vi "PollReceiveQueueNoSemaphore.vi"(8 "error in (no error)":errorcluster, 10 "waiting time ms (-1: forever)":i32=10, 11 "queue cluster":T1) -> (1 "receive queue error out":errorcluster, 2 "# elements in queue":i32, 3 "receive queue":refnum<queue>)   [LabVIEW 2014]
uses:
  typedefs/QueueCluster.ctl
  typedefs/clientStatus.ctl
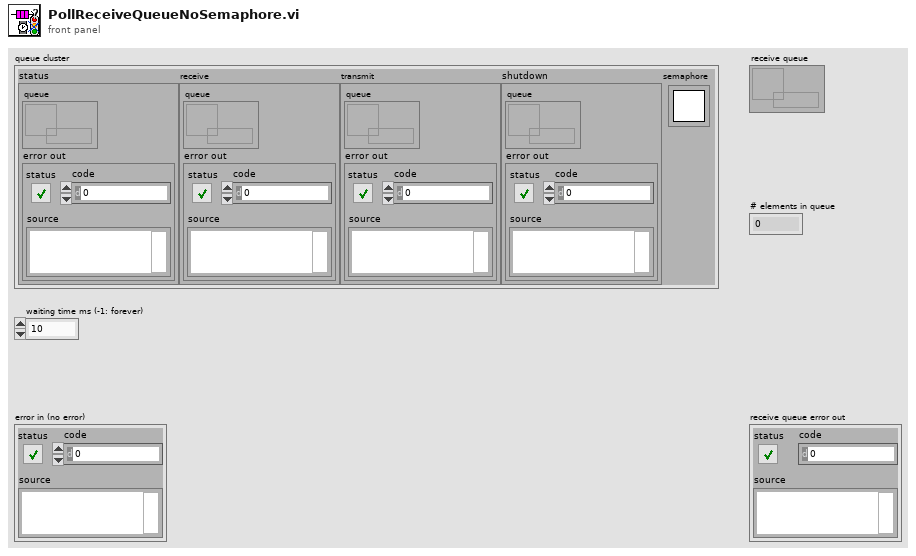
[diagram p1: front panel]
types:
  T1 = typedef "QueueCluster.ctl" = cluster{"status":cluster{"queue":refnum<queue>, "error out":errorcluster}, "receive":cluster{"queue":refnum<queue>, "error out":errorcluster}, "transmit":cluster{"queue":refnum<queue>, "error out":errorcluster}, "shutdown":cluster{"queue":refnum<queue>, "error out":errorcluster}, "semaphore":T2}
  T2 = typedef "Semaphore RefNum" = refnum<k1>
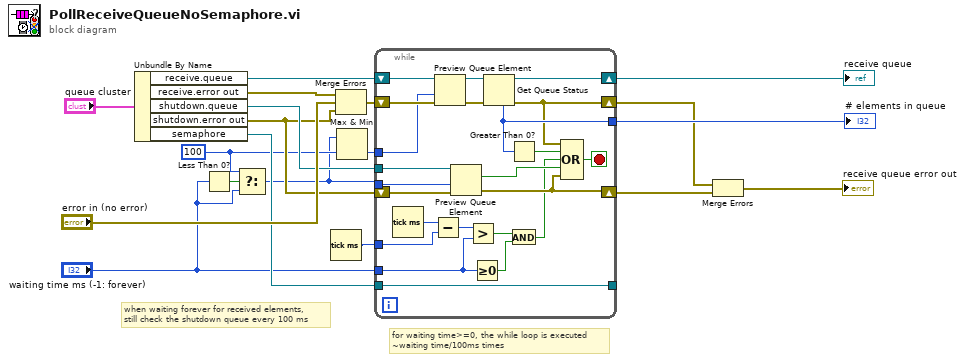
[diagram p0: block diagram]
diagram:
  w2 = 100 ("t")
  # "for waiting time>=0, the while loop is executed\n~waiting time/100ms times"
  # "when waiting forever for received elements,\nstill check the shutdown queue every 100 ms"
  n1 = Unbundle By Name("queue cluster") -> ("receive.queue"=w13:refnum<queue>, "receive.error out"=w16:errorcluster, "shutdown.queue"=w11:refnum<queue>, "shutdown.error out"=w6:errorcluster, "semaphore"=w10:T2)
  n2 = Less Than 0?(x="waiting time ms (-1: forever)") -> (x < 0?=w5:bool)
  n3 = Select(t=w2, s=w5, f="waiting time ms (-1: forever)") -> (s? t:f=w1:i32)
  n4 = Tick Count (ms)() -> (millisecond timer value=w18:u32)
  n5 = Merge Errors(w16, "error in (no error)", w6) -> (w15:errorcluster)
  n6 = Max & Min(x=w1, y=w2) -> (min(x,y)=w3:i32)  [unwired: 1 out]
  n7 = while {
    tunnel: [w40] -> w19
    shift-right: [w42] -> w14
    shift-left: w13 -> [w24]
    shift-right: [w34] -> w8
    shift-left: w15 -> [w22]
    tunnel: w18 -> [w38]
    tunnel: "waiting time ms (-1: forever)" -> [w29]
    tunnel: [w35] -> _
    tunnel: w10 -> [w35]
    tunnel: w11 -> [w33]
    shift-right: [w30] -> w9
    shift-left: w6 -> [w31]
    tunnel: w1 -> [w25]
    tunnel: w3 -> [w20]
    stop <- w36 stop-if-true
    n8 = Tick Count (ms)() -> (millisecond timer value=w39:u32)
    n9 = Subtract(x=w39, y=w38) -> (x-y=w37:u32)
    n10 = Preview Queue Element(queue=w24, timeout in ms (-1)=w20, error in (no error)=w22) -> (queue out=w23:refnum<queue>, error out=w21:errorcluster)  [unwired: 2 out]
    n11 = Preview Queue Element(queue=w33, timeout in ms (-1)=w25, error in (no error)=w31) -> (element=w32:bool, error out=w30:errorcluster)  [unwired: 2 out]
    n12 = Greater?(x=w37, y=w29) -> (0:w27:bool)
    n13 = Greater Or Equal To 0?(x=w29) -> (x >= 0?=w28:bool)
    n14 = Get Queue Status(queue=w23, error in (no error)=w21) -> (queue out=w42:refnum<queue>, error out=w34:errorcluster, # elements in queue=w40:i32)  [unwired: 1 in, 5 out]
    n15 = Greater Than 0?(x=w40) -> (x > 0?=w41:bool)
    n16 = And(x=w27, y=w28) -> (x .and. y?=w26:bool)
    n17 = Compound Arithmetic op=OR(w34, w41, w26, w32, w30) -> (w36:bool)
  }
  "# elements in queue" <- w19
  "receive queue" <- w14
  n18 = Merge Errors(w8, w9) -> (→"receive queue error out":errorcluster)
